vi "Init Menu.vi"(8 "error in (no error)":errorcluster) -> (0 "error out":errorcluster)   [LabVIEW 2019, in "Menu Launcher Module.lvlib"]
doc: "Init Menu With the Menu File\n_____\nCreated using Delacor QMH Event Scripter 5.0.0.112."
uses:
  Menu Launcher Module.lvlib
  Init Menu Argument--cluster.ctl
  Utility/Controls/Menu_Configuration.ctl
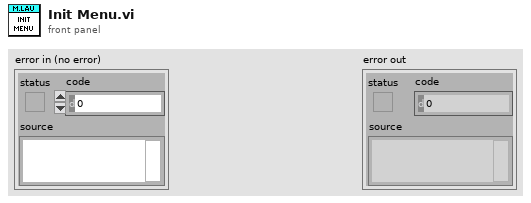
[diagram p1: front panel]
types:
  T1 = typedef "Menu Launcher Module.lvlib/Init Menu Argument--cluster.ctl" = cluster{"Menu_Configuration":T2, "Module ID":i32}
  T2 = typedef "Menu_Configuration.ctl" = cluster{"Button_Label_Color":u32, "Button_Color_On":u32, "Button_Color_Off":u32, "Panel_Color":u32, "Extend_Sub_Menu_Icon":path, "Root_Menu_Data":cluster{"Button_Icon":path, "Button_Label":string, "Sub_Menu_Data":cluster{"Button_Icon":path, "Button_Label":string, "Child_Menu_Data":cluster{"Button_Icon":path, "Button_Label":string}[]}[]}[]}
  T3 = typedef "Menu Launcher Module.lvlib/Request Events--cluster.ctl" = cluster{"Stop Module":refnum<user-event>, "Show Panel":refnum<user-event>, "Hide Panel":refnum<user-event>, "Get Module Execution Status":refnum<user-event>, "Show Diagram":refnum<user-event>, "Init Menu Configuration":refnum<user-event>, "Init Menu":refnum<user-event>, "Change Menu Configure":refnum<user-event>, "Launch Menu":refnum<user-event>, "Close Menu":refnum<user-event>}
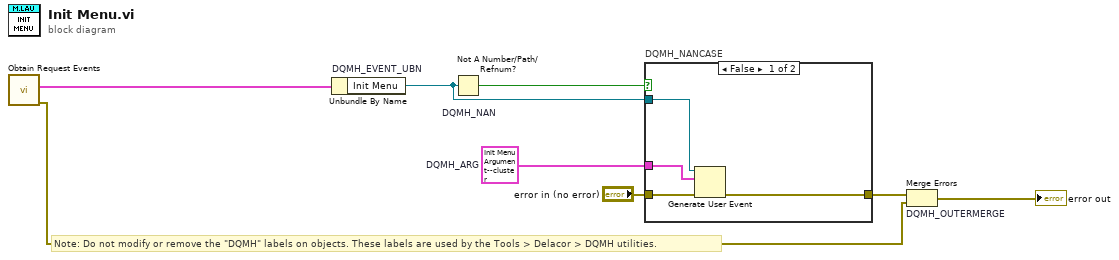
[diagram p0: block diagram]
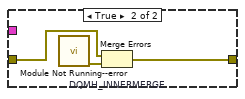
[diagram p2: hidden frame]
diagram:
  w1 = T1 {"Menu_Configuration"={"Button_Label_Color"=2344, "Button_Color_On"=5654, "Button_Color_Off"=2344, "Panel_Color"=2344, "Extend_Sub_Menu_Icon"=path "C:/Users/SyncSols-4/Desktop/Icon/Accept-icon.png", "Root_Menu_Data"=[{"Button_Icon"=path "C:/Users/SyncSols-4/Desktop/Icon/Accept-icon.png", "Button_Label"="Test", "Sub_Menu_Data"=[{"Button_Icon"=path "C:/Users/SyncSols-4/Desktop/Icon/floppy-icon.png", "Button_Label"="Save", "Child_Menu_Data"=[]}, {"Button_Icon"=path "C:/Users/SyncSols-4/Desktop/Icon/folder-icon1.png", "Button_Label"="Folder", "Child_Menu_Data"=[]}, {"Button_Icon"=path "C:/Users/SyncSols-4/Desktop/Icon/delete-icon.png", "Button_Label"="Delete", "Child_Menu_Data"=[{"Button_Icon"=path "C:/Users/SyncSols-4/Desktop/Icon/add-icon.png", "Button_Label"="Add"}, {"Button_Icon"=path "C:/Users/SyncSols-4/Desktop/Icon/Stop-red-icon.png", "Button_Label"="Stop"}]}]}, {"Button_Icon"=path "C:/Users/SyncSols-4/Desktop/Icon/add-key-icon.png", "Button_Label"="Key", "Sub_Menu_Data"=[]}, {"Button_Icon"=path "C:/Users/SyncSols-4/Desktop/Icon/Categories-preferences-system-icon.png", "Button_Label"="Setting", "Sub_Menu_Data"=[]}]}, "Module ID"=0}  # DQMH_ARG
  # "Note: Do not modify or remove the \"DQMH\" labels on objects. These labels are used by the Tools > Delacor > DQMH utilities."
  n1 = call "Obtain Request Events.vi"() -> ("error out"=w3:errorcluster, "Menu Launcher Module Request Events"=w2:T3)  [unwired: 10 in]
  n2 = Unbundle By Name "DQMH_EVENT_UBN"(w2) -> ("Init Menu"=w5:refnum<user-event>)
  n3 = Not A Number/Path/Refnum? "DQMH_NAN"(number/path/refnum=w5) -> (NaN/Path/Refnum?=w6:bool)
  n4 = case "DQMH_NANCASE" shown="False" w6 {
    tunnel: "error in (no error)" -> [w12 w15]
    tunnel: [w11 w14] -> w4
    tunnel: w5 -> [w10 _]
    tunnel: w1 -> [w9 _]
    frame False {
      n5 = Generate User Event(user event=w10, event data cluster=w9, error in=w12) -> (error out=w11:errorcluster)  [unwired: 1 in, 1 out]
    }
    frame True {
      n6 = call "Module Not Running--error.vi"() -> ("error out"=w13:errorcluster)  [unwired: 11 in]
      n7 = Merge Errors "DQMH_INNERMERGE"(w15, w13) -> (w14:errorcluster)
    }
  }
  n8 = Merge Errors "DQMH_OUTERMERGE"(w4, w3) -> (→"error out":errorcluster)
